vi "SpeedTokenizer.vi"(8 "error in (no error)":errorcluster, 11 "string 2":string) -> (0 "error out":errorcluster, 3 "Array 2":string[](array[string]))   [LabVIEW 2019, in "PathTokenizer.lvclass"]
uses:
  PathTokenizer.lvclass
  <vilib>/Utility/error.llb/whitespace.ctl
  <vilib>/regexp/Match Regular Expression.xnode
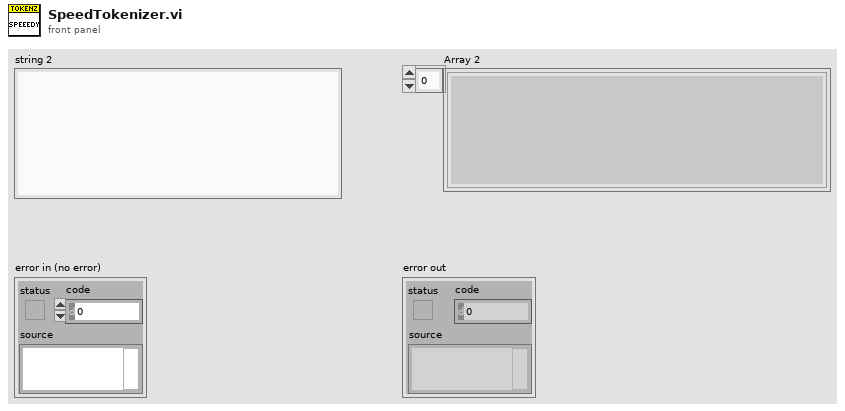
[diagram p1: front panel]
types:
  T1 = typedef "whitespace.ctl" = u16
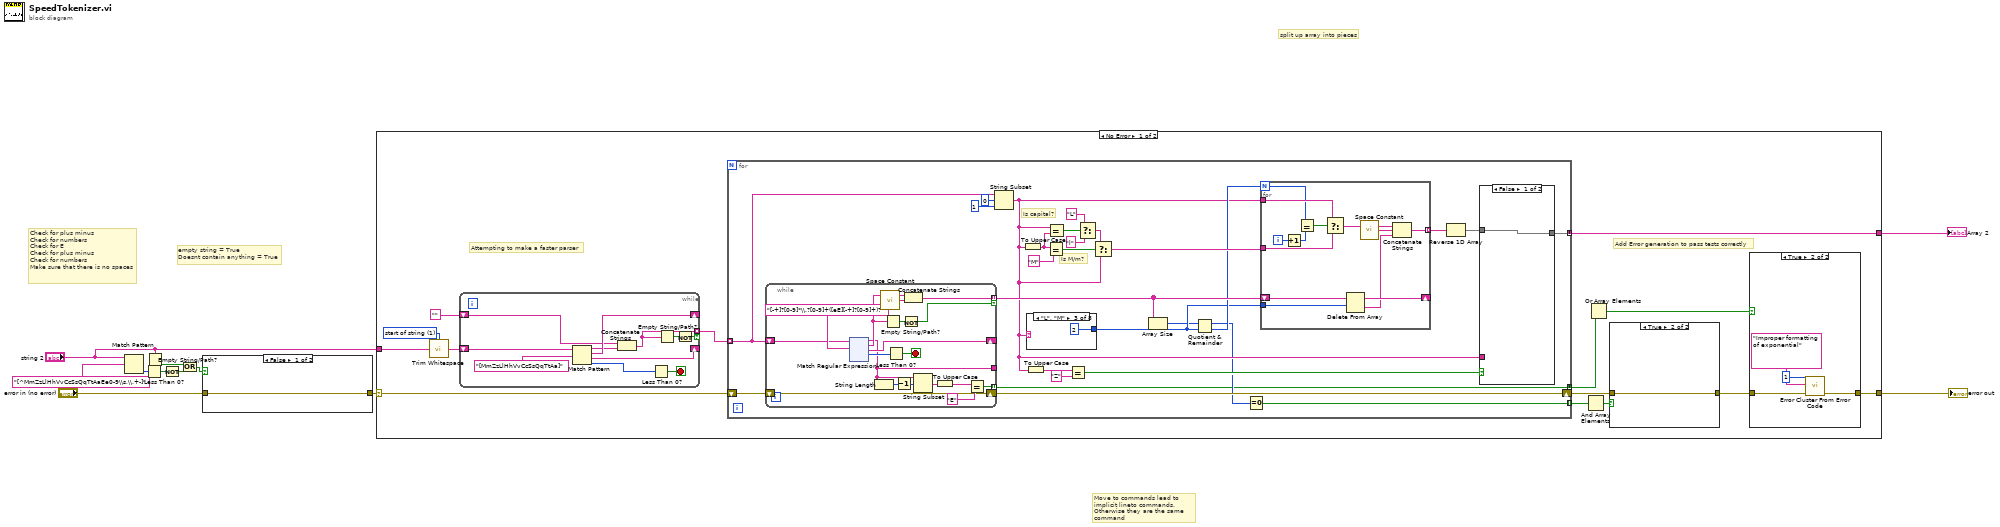
[diagram p0: block diagram]
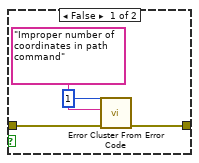
[diagram p3: hidden frame]
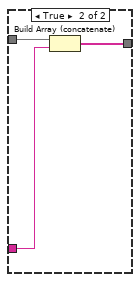
[diagram p4: hidden frame]
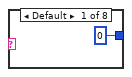
[diagram p5: hidden frame]
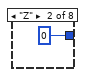
[diagram p6: hidden frame]
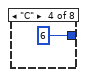
[diagram p7: hidden frame]
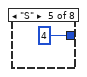
[diagram p8: hidden frame]
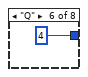
[diagram p9: hidden frame]
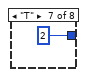
[diagram p10: hidden frame]
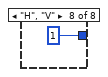
[diagram p11: hidden frame]
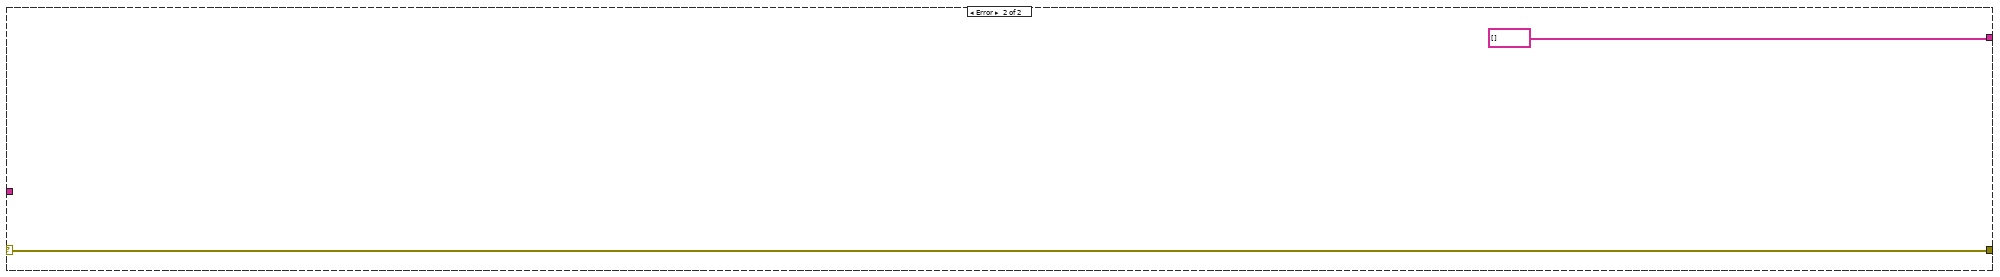
[diagram p12: hidden frame]
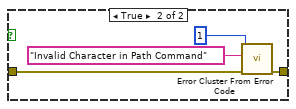
[diagram p13: hidden frame]
diagram:
  # "empty string = True\nDoesnt contain anything = True"
  # "Move to commands lead to implicit lineto commands. Otherwise they are the same command"
  # "split up array into pieces"
  # "Check for plus minus\nCheck for numbers\nCheck for E\nCheck for plus minus\nCheck for numbers\nMake sure that there is no spaces"
  n1 = Match Pattern(string="string 2", regular expression="[^MmZzLlHhVvCcSsQqTtAaEe0-9\\s,\\.+-]") -> (offset past match=w9:i32)  [unwired: 1 in, 3 out]
  n2 = Less Than 0?(x=w9) -> (x < 0?=w4:bool)
  n3 = Empty String/Path?(string/path="string 2") -> (empty?=w2:bool)
  n4 = Not(x=w4) -> (.not. x?=w3:bool)
  n5 = Or(x=w2, y=w3) -> (x .or. y?=w1:bool)
  n6 = case shown="False" w1 {
    tunnel: "error in (no error)" -> [w12 w14]
    tunnel: [w12 w13] -> w6
    frame False {
    }
    frame True {
      n7 = call <vilib>:"Error Cluster From Error Code.vi"("error in (no error)"=w14, "error message (\"\")"="Invalid Character in Path Command" ("error message (\"\")"), "error code (0)"=1) -> ("error out"=w13:errorcluster)  [unwired: 6 in]
    }
  }
  n8 = case shown="No Error" w6 {
    selector: w6 -> [w24 w236]
    tunnel: [w26 string[] []] -> w11
    tunnel: [w18 w236] -> w10
    tunnel: "string 2" -> [w25 _]
    frame No Error {
      w29 = T1 1 items=["both", "start of string", "end of string"] ("location (both)")
      # "Add Error generation to pass tests correctly"
      # "Attempting to make a faster parser"
      n9 = call <vilib>:"Trim Whitespace.vi"("string"=w25, "location (both)"=w29) -> ("trimmed string"=w30:string)
      n10 = while {
        shift-right: [w230] -> _
        shift-left: w30 -> [w235]
        shift-right: [w233] -> _
        shift-left: "" -> [w231]
        tunnel: [w227] -> w28 mode=indexing if=w225
        stop <- w229 stop-if-true
        n11 = Match Pattern(string=w235, regular expression="[MmZzLlHhVvCcSsQqTtAa]") -> (before substring=w232:string, match substring=w233:string, after substring=w230:string, offset past match=w228:i32)  [unwired: 1 in]
        n12 = Concatenate Strings(w231, w232) -> (w227:string)
        n13 = Less Than 0?(x=w228) -> (x < 0?=w229:bool)
        n14 = Empty String/Path?(string/path=w227) -> (empty?=w226:bool)
        n15 = Not(x=w226) -> (.not. x?=w225:bool)
      }
      n16 = for {
        tunnel: w28 -> [w65] mode=indexing
        tunnel: [w51] -> w26 mode=concatenating
        shift-right: [w62] -> w21
        shift-left: w24 -> [w63]
        tunnel: [w42] -> w23 mode=indexing
        tunnel: [w41] -> w20 mode=concatenating
        # "Is M/m?"
        # "Is capital?"
        n17 = while {
          shift-right: [w108] -> _
          shift-left: w65 -> [w109]
          tunnel: [w102] -> w49 mode=indexing if=w101
          shift-right: [w94] -> w62
          shift-left: w63 -> [w94]
          tunnel: [w93] -> _
          tunnel: [w95] -> w41 mode=indexing
          stop <- w106 stop-if-true
          n18 = xnode "Match Regular Expression"("input string"=w109, "regular expression"="[-+]?[0-9]*\\.?[0-9]+([eE][-+]?[0-9]+)?") -> ("before match"=w93:string, "whole match"=w103:string, "after match"=w108:string, "offset past match"=w107:i32)  [unwired: 4 in, 1 out]
          n19 = String Length(string=w93) -> (length=w100:i32)
          n20 = call <vilib>:"Space Constant.vi"() -> ("String"=w104:string)
          n21 = Empty String/Path?(string/path=w103) -> (empty?=w105:bool)
          n22 = Less Than 0?(x=w107) -> (x < 0?=w106:bool)
          n23 = Decrement(x=w100) -> (x-1=w97:i32)
          n24 = Not(x=w105) -> (.not. x?=w101:bool)
          n25 = Concatenate Strings(w103, w104) -> (w102:string)
          n26 = String Subset(string=w93, offset (0)=w97) -> (substring=w99:string)  [unwired: 1 in]
          n27 = To Upper Case(1:w99) -> (0:w96:string)
          n28 = Equal?(x=w96, y="E") -> (x = y?=w95:bool)
        }
        n29 = String Subset(string=w65, offset (0)=0, length (rest)=1 ("length (rest)")) -> (substring=w45:string)
        n30 = To Upper Case(1:w45) -> (0:w59:string)
        n31 = case shown="\"L\", \"M\"" w45 {
          tunnel: [0 0 2 6 4 4 2 1] -> w46
          frame Default {
            # "There was an error handler here for unsupported command type"
          }
          frame "Z" {
          }
          frame "L", "M" {
          }
          frame "C" {
          }
          frame "S" {
          }
          frame "Q" {
          }
          frame "T" {
          }
          frame "H", "V" {
          }
        }
        n32 = To Upper Case(1:w45) -> (0:w54:string)
        n33 = Equal?(x=w59, y="M") -> (x = y?=w61:bool)
        n34 = Equal?(x=w45, y=w59) -> (x = y?=w58:bool)
        n35 = Equal?(x=w54, y="Z") -> (x = y?=w50:bool)
        n36 = Select(t="L", s=w58, f="l") -> (s? t:f=w55:string)
        n37 = Select(t=w55, s=w61, f=w45) -> (s? t:f=w48:string)
        n38 = Array Size(array=w49) -> (size(s)=w44:i32)
        n39 = Quotient & Remainder(x=w44, y=w46) -> (x-y*floor(x/y)=w43:i32, floor(x/y)=w47:i32)
        n40 = Equal To 0?(x=w43) -> (x = 0?=w42:bool)
        n41 = for {
          N: w47 -> [w72]
          tunnel: w46 -> [w82]
          shift-right: [w84] -> _
          shift-left: w49 -> [w83]
          tunnel: [w79] -> w64 mode=indexing
          tunnel: w45 -> [w76]
          tunnel: w48 -> [w78]
          i -> [w73]
          n42 = Increment(x=w73) -> (x+1=w74:i32)
          n43 = Equal?(x=w72, y=w74) -> (x = y?=w75:bool)
          n44 = Select(t=w76, s=w75, f=w78) -> (s? t:f=w77:string)
          n45 = Delete From Array(array=w83, length=w82) -> (deleted portion=w80:string[], array with subset deleted=w84:string[])  [unwired: 1 in]
          n46 = call <vilib>:"Space Constant.vi"() -> ("String"=w81:string)
          n47 = Concatenate Strings(w77, w81, w80) -> (w79:string)
        }
        n48 = Reverse 1D Array(array=w64) -> (reversed array=w52:string[])
        n49 = case shown="False" w50 {
          tunnel: w52 -> [w68 w70]
          tunnel: [w68 w69] -> w51
          tunnel: w45 -> [_ w71]
          frame False {
          }
          frame True {
            n50 = Build Array (concatenate)(w70, w71) -> (w69:string[])
          }
        }
      }
      n51 = And Array Elements(Boolean array=w23) -> (logical AND=w22:bool)
      n52 = Or Array Elements(Boolean array=w20) -> (logical OR=w17:bool)
      n53 = case shown="True" w22 {
        tunnel: w21 -> [w39 w40]
        tunnel: [w38 w40] -> w19
        frame False {
          n54 = call <vilib>:"Error Cluster From Error Code.vi"("error in (no error)"=w39, "error message (\"\")"="Improper number of coordinates in path command" ("error message (\"\")"), "error code (0)"=1) -> ("error out"=w38:errorcluster)  [unwired: 6 in]
        }
        frame True {
        }
      }
      n55 = case shown="True" w17 {
        tunnel: w19 -> [w31 w35]
        tunnel: [w31 w34] -> w18
        frame False {
        }
        frame True {
          n56 = call <vilib>:"Error Cluster From Error Code.vi"("error in (no error)"=w35, "error message (\"\")"="Improper formatting of exponential" ("error message (\"\")"), "error code (0)"=1) -> ("error out"=w34:errorcluster)  [unwired: 6 in]
        }
      }
    }
    frame Error {
    }
  }
  "error out" <- w10
  "Array 2" <- w11
